vi "Step 1.vi"(8 "error in (no error)":errorcluster, 11 "HeatUp Data in":string[][](array[string])) -> (0 "error out":errorcluster, 1 "Water Heater Type":T1, 2 "Time":bool, 3 "Gallon @ Compressor ON\nOr Time Value (Minutes)":dbl, 4 "HeatUp Data in 2":string[][](array[string]))   [LabVIEW 2016]
uses:
  Type Definitions/HEWH_Type.ctl
  <vilib>/Utility/error.llb/DialogType.ctl
panel:
  out "Second Difference":dbl
  out "Time at 10.75":dbl
  out "transposed array":string[][](array[string])
  out "Index of 10.75":i32
  out "Time":dbl
  # "Data with Stripped Header"
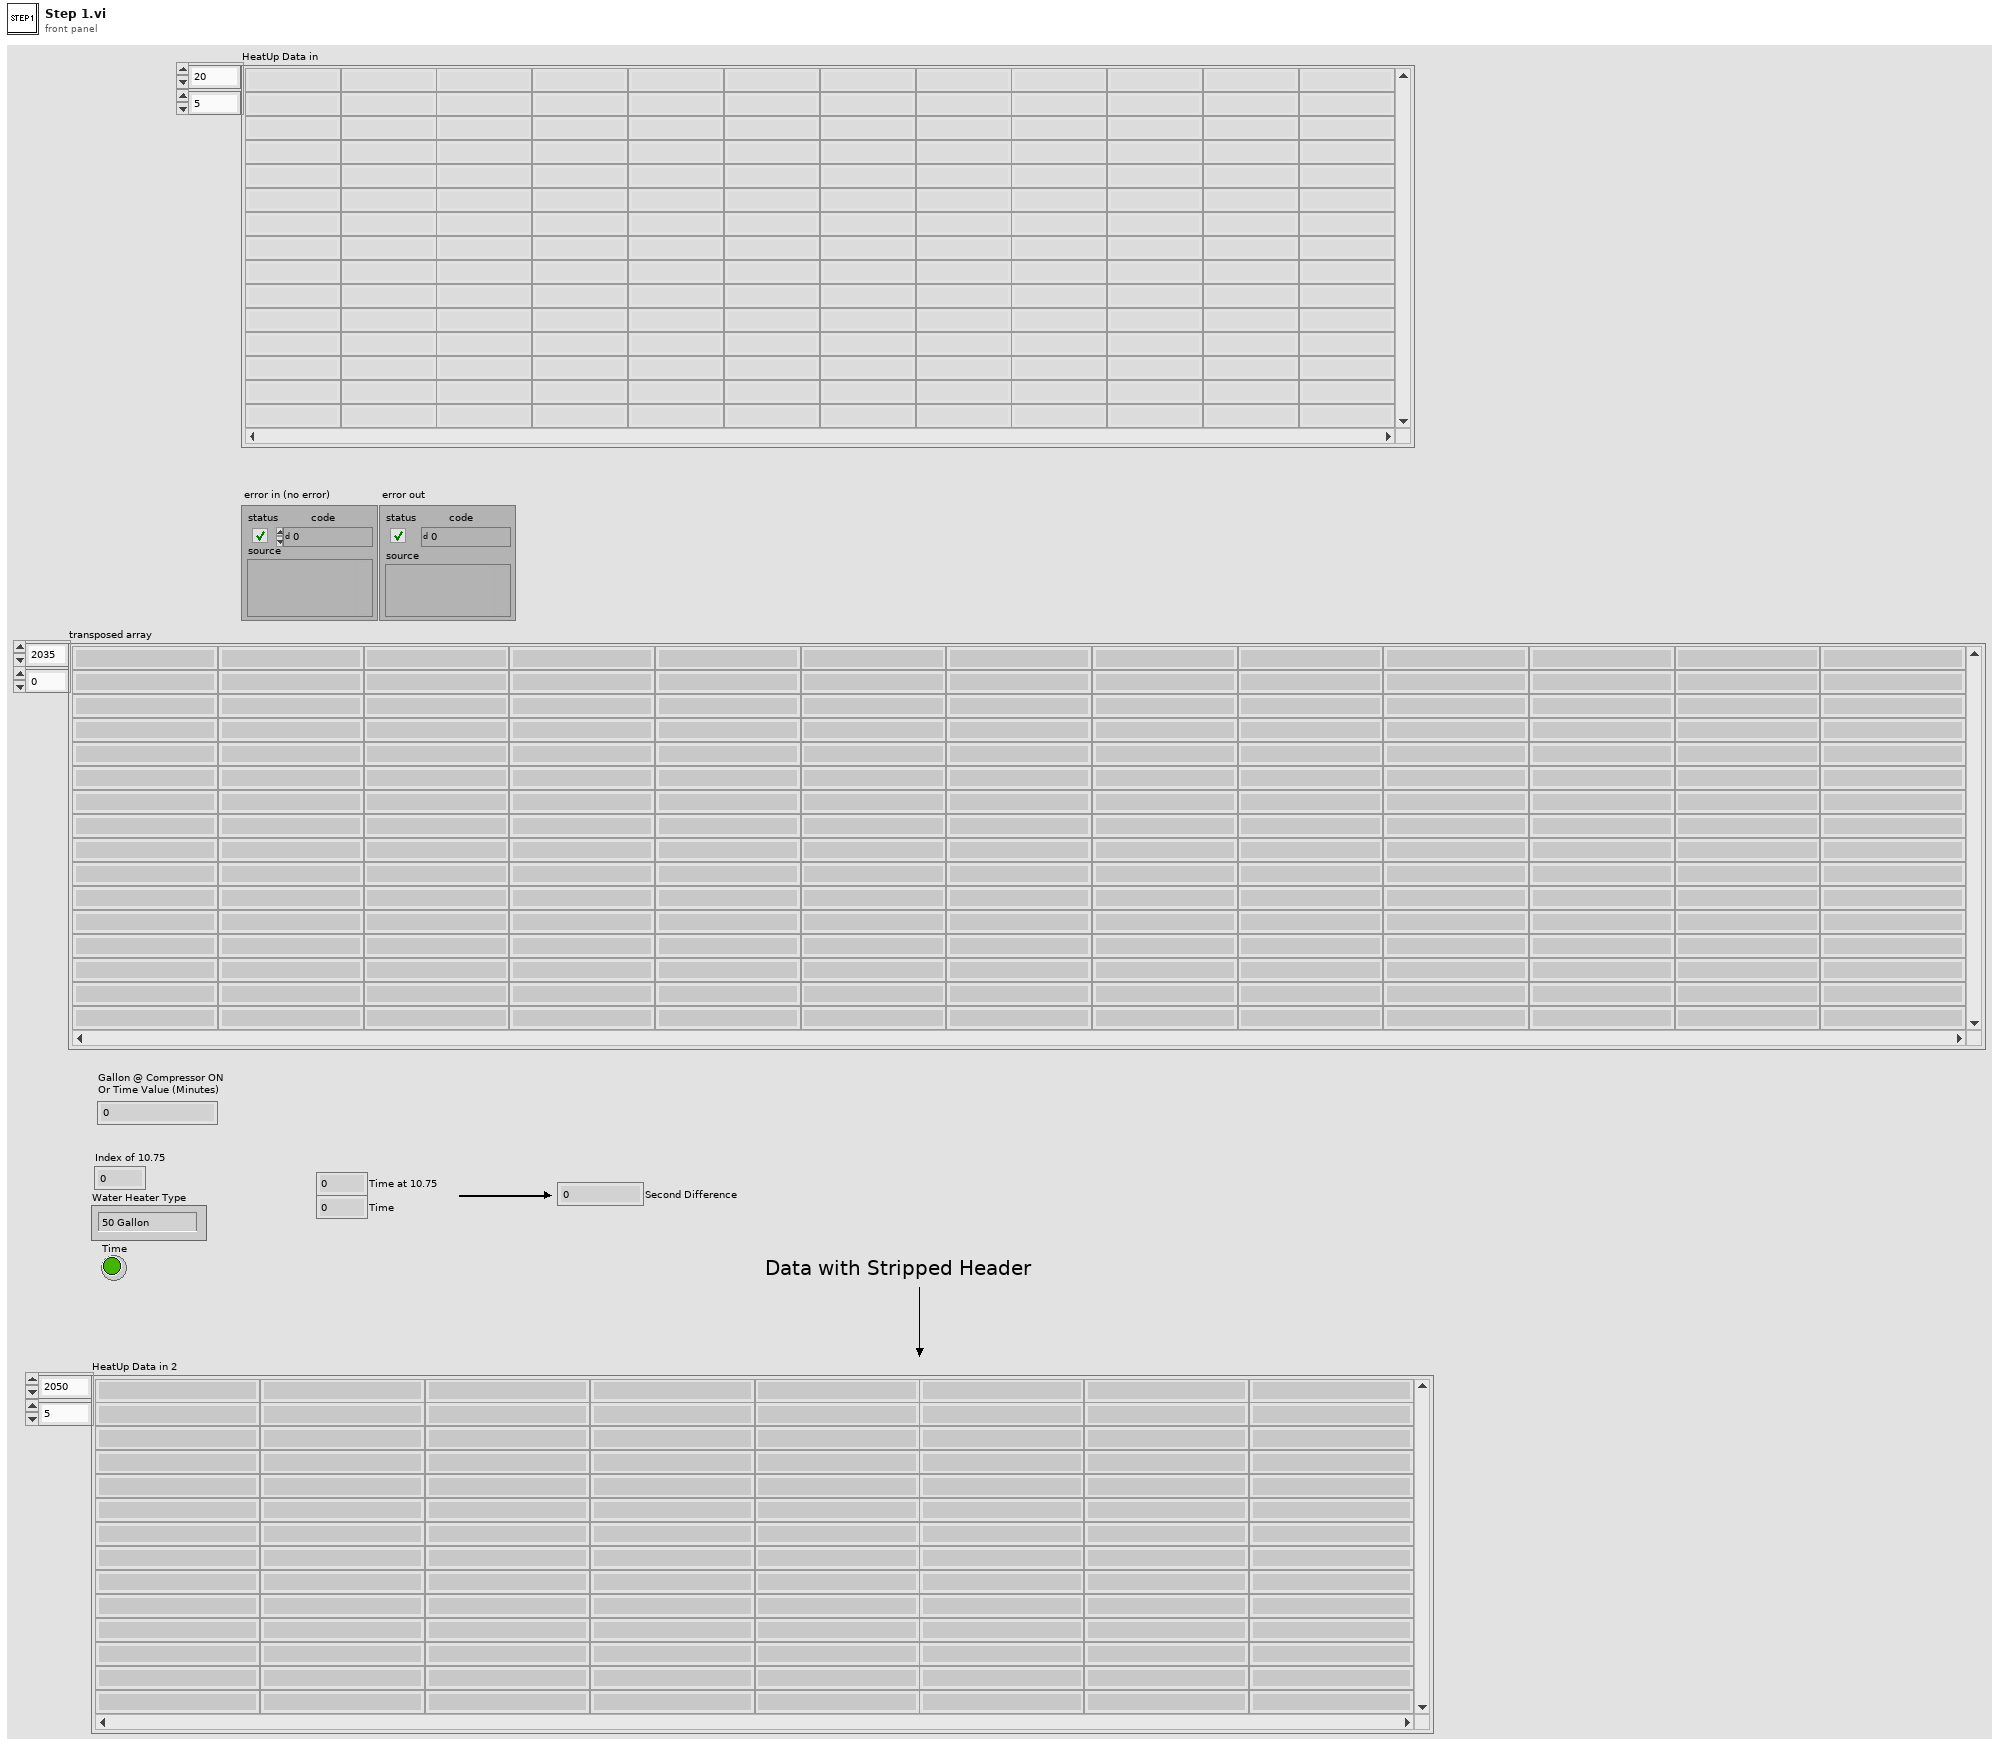
[diagram p1: front panel]
types:
  T1 = typedef "HEWH_Type.ctl" = enum16{"50 Gallon", "80 Gallon"}
  T2 = typedef "DialogType.ctl" = u16
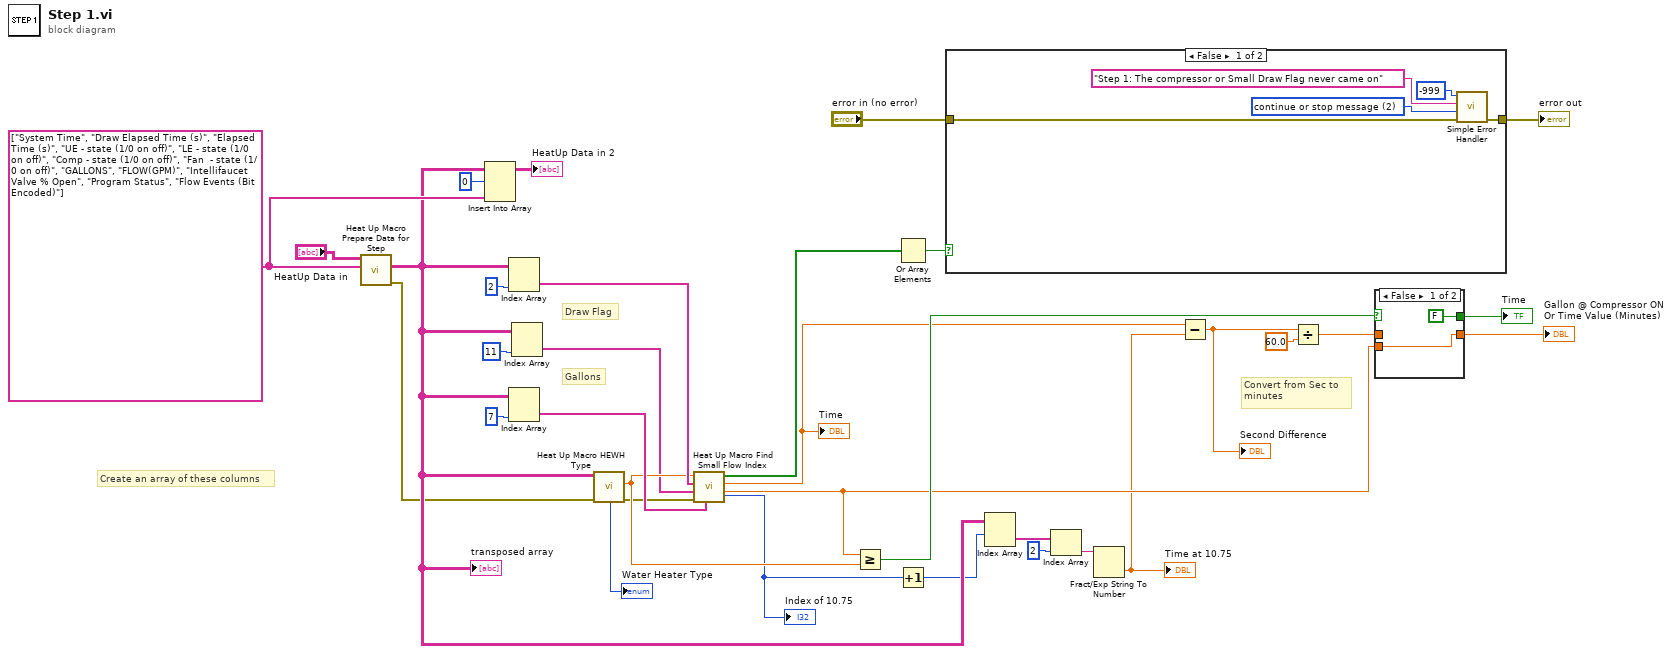
[diagram p0: block diagram]
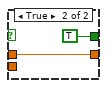
[diagram p3: hidden frame]
diagram:
  w11 = string[] ["System Time", "Draw Elapsed Time (s)", "Elapsed Time (s)", "UE - state (1/0 on off)", "LE - state (1/0 on off)", "Comp - state (1/0 on off)", "Fan  - state (1/0 on off)", "GALLONS", "FLOW(GPM)", "Intellifaucet Valve % Open", "Program Status", "Flow Events (Bit Encoded)"]
  # "Draw Flag"
  # "Gallons"
  # "Convert from Sec to\nminutes"
  # "Create an array of these columns"
  n1 = call "Heat Up Macro Prepare Data for Step.vi"("Columns Too Search For"=w11, "HeatUp Raw Data Input"="HeatUp Data in") -> ("Error Out"=w2:errorcluster, "Heat Up Data with Only Selected Columns"=w6:string[][])  [unwired: 8 in]
  "transposed array" <- w6
  n2 = Insert Into Array(array=w6, index (row)=0, new element=w11) -> (→"HeatUp Data in 2":string[][])  [unwired: 1 in]
  n3 = Index Array(array=w6, index (col)=2 ("disabled index (col)")) -> (element=w26:string[])  [unwired: 1 in]
  n4 = Index Array(array=w6, index (col)=7 ("disabled index (col)")) -> (element=w30:string[])  [unwired: 1 in]
  n5 = Index Array(array=w6, index (col)=11 ("disabled index (col)")) -> (element=w9:string[])  [unwired: 1 in]
  n6 = call "Heat Up Macro HEWH Type.vi"("Error In"=w2, "Heat Up Data with Only Selected Columns"=w6) -> ("Error Out"=w1:errorcluster, "Gallon Target"=w24:dbl, "Water Heater Type"=→"Water Heater Type":T1)  [unwired: 7 in]
  n7 = call "Heat Up Macro Find Small Flow Index.vi"("Gallons"=w30, "Error In"=w1, "Draw Flag Column"=w9, "Elapsed Time"=w26, "Gallon Target"=w24) -> ("Gallons"=w28:dbl, "Time"=w21:dbl, "Error Array. If all false"=w8:bool[], "Numeric"=w5:i32)  [unwired: 2 in, 1 out]
  "Time" <- w21
  "Index of 10.75" <- w5
  n8 = Greater Or Equal?(x=w28, y=w24) -> (x >= y?=w29:bool)
  n9 = Or Array Elements(Boolean array=w8) -> (logical OR=w7:bool)
  n10 = Increment(x=w5) -> (x+1=w4:i32)
  n11 = case shown="False" w7 {
    tunnel: "error in (no error)" -> [w38 w39]
    tunnel: [w37 w39] -> w13
    frame False {
      w36 = T2 2 items=["no dialog", "OK message", "continue or stop message", "OK message + warnings", "continue/stop + warnings"] ("type of dialog (OK msg:1)")
      n12 = call <vilib>:"Simple Error Handler.vi"("error code (no error:0)"=-999, "error source (\" \")"="Step 1: The compressor or Small Draw Flag never came on" ("error source (\" \")"), "type of dialog (OK msg:1)"=w36, "error in (no error)"=w38) -> ("error out"=w37:errorcluster)  [unwired: 1 in, 4 out]
    }
    frame True {
    }
  }
  "error out" <- w13
  n13 = Index Array(array=w6, index (row)=w4) -> (element=w23:string[])  [unwired: 1 in]
  n14 = Index Array(array=w23, index=2) -> (element=w20:string)
  n15 = Fract/Exp String To Number(string=w20) -> (number=w19:dbl)  [unwired: 3 in, 1 out]
  "Time at 10.75" <- w19
  n16 = Subtract(x=w21, y=w19) -> (x-y=w18:dbl)
  "Second Difference" <- w18
  n17 = Divide(x=w18, y=60.0) -> (x/y=w16:dbl)
  n18 = case shown="False" w29 {
    tunnel: w28 -> [w41 _]
    tunnel: [w41 w43] -> w27
    tunnel: w16 -> [_ w43]
    tunnel: [FALSE TRUE] -> w15
    frame False {
    }
    frame True {
    }
  }
  "Gallon @ Compressor ON\nOr Time Value (Minutes)" <- w27
  "Time" <- w15
